vi "Wczytaj_wzmocnienia_analogowe_INI.vi"(8 "error in (no error)":errorcluster, 11 "Path ini":path=path "D:/Marek/Documents/LabVIEW SVN/Rudpol2/Konfiguracja/Karty_AI.ini") -> (0 "error out":errorcluster, 2 "Wzmocnienia":dbl[][](array[numeric]))   [LabVIEW 2013]
doc: "Wczytuje wzmocnienia dla kazdego kana³u analogowego\nz pliku konfiguracyjnego Karty_AI.ini"
uses:
  <vilib>/Utility/config.llb/NI_LVConfig.lvlib
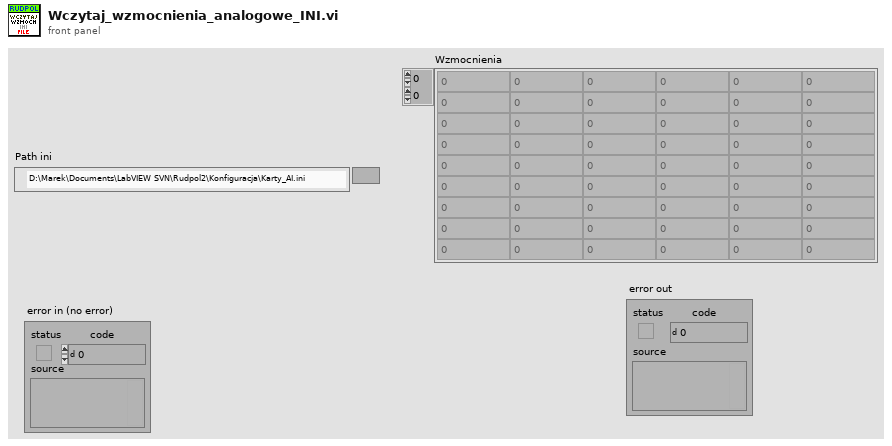
[diagram p1: front panel]
types:
  T1 = typedef "NI_LVConfig.lvlib/Config Data RefNum.ctl" = refnum<k1>
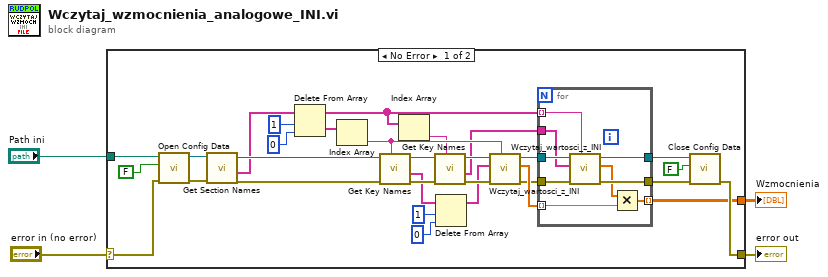
[diagram p0: block diagram]
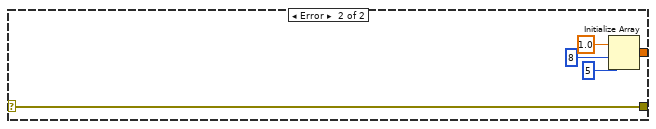
[diagram p2: hidden frame]
diagram:
  n1 = case shown="No Error" "error in (no error)" {
    selector: "error in (no error)" -> [w34 w49]
    tunnel: [w28 w49] -> w3
    tunnel: "Path ini" -> [w35 _]
    tunnel: [w5 w45] -> w1
    frame No Error {
      n2 = call <vilib>:"Open Config Data.vi"("error in (no error)"=w34, "create file if necessary (T)"=FALSE, "configuration file path"=w35) -> ("error out"=w31:errorcluster, "refnum"=w32:T1)  [unwired: 6 in, 1 out]
      n3 = call <vilib>:"Get Section Names.vi"("error in (no error)"=w31, "refnum"=w32) -> ("error out"=w29:errorcluster, "section names"=w24:string[], "refnum out"=w30:T1)  [unwired: 7 in]
      n4 = Delete From Array ("section names")(array=w24, length=1, index=0) -> (deleted portion=w23:string[], array with subset deleted=w11:string[])
      n5 = Index Array(array=w23) -> (element=w17:string)  [unwired: 1 in]
      n6 = call <vilib>:"Get Key Names.vi"("section"=w17, "error in (no error)"=w29, "refnum"=w30) -> ("error out"=w16:errorcluster, "key names"=w8:string[], "refnum out"=w15:T1)  [unwired: 5 in, 1 out]
      n7 = Index Array(array=w11) -> (element=w12:string)  [unwired: 1 in]
      n8 = call <vilib>:"Get Key Names.vi"("section"=w12, "error in (no error)"=w16, "refnum"=w15) -> ("error out"=w14:errorcluster, "key names"=w6:string[], "refnum out"=w13:T1)  [unwired: 5 in, 1 out]
      n9 = Delete From Array(array=w8, length=1, index=0) -> (array with subset deleted=w7:string[])  [unwired: 1 out]
      n10 = call "Wczytaj_wartosci_z_INI.vi"("Section"=w17, "error in (no error)"=w14, "key names"=w7, "refnum"=w13) -> ("error out"=w21:errorcluster, "Array"=w22:dbl[], "refnum out"=w20:T1)  [unwired: 5 in]
      n11 = for {
        tunnel: w22 -> [w37] mode=indexing
        tunnel: w21 -> [w44]
        tunnel: w20 -> [w43]
        tunnel: [w41] -> w19
        tunnel: w11 -> [w40] mode=indexing
        tunnel: w6 -> [w39]
        tunnel: [w42] -> w18
        tunnel: [w36] -> w5 mode=indexing
        n12 = call "Wczytaj_wartosci_z_INI.vi"("Section"=w40, "error in (no error)"=w44, "key names"=w39, "refnum"=w43) -> ("error out"=w42:errorcluster, "Array"=w38:dbl[], "refnum out"=w41:T1)  [unwired: 5 in]
        n13 = Multiply(x=w38, y=w37) -> (x*y=w36:dbl[])
      }
      n14 = call <vilib>:"Close Config Data.vi"("error in (no error)"=w18, "write file if changed (T)"=FALSE, "refnum"=w19) -> ("error out"=w28:errorcluster)  [unwired: 7 in, 1 out]
    }
    frame Error {
      n15 = Initialize Array(1.0 ("element"), 8 ("dimension size"), 5 ("dimension size")) -> (w45:dbl[][])
    }
  }
  "error out" <- w3
  "Wzmocnienia" <- w1
